vi "newTest_interface.vi"(0 "Daten":T1={"Report.lvclass"=refnum, "Norm"="", "last State"=enum."Initialize", "Norm ID"=0, "parameter"=[], "EMTestCWS500N.lvclass"=refnum, "CEG4500.lvclass"=refnum, "Tektronix RSA5106A.lvclass"=refnum, "erfolgreich"=FALSE, "log"="", "Kommentar"="", "Device Enum"=enum."emTestCWS500N", "Test Enum"=enum."HF-Felder", "debug"=FALSE, "tab"=enum."Hauptmenü", "ESD Pistol.lvclass"=refnum, "SubPnl Refnum"=refnum, "TabCtl Refnum"=refnum, "ButtonsEinblenden?"=FALSE}, 1 "Test in":refnum<class "Test.lvclass">, 3 "error in (no error)":errorcluster, 4 "VI Refnum":refnum<vi>) -> (7 "Test.lvclass":refnum<class "Test.lvclass">, 8 "abbrechen":bool, 10 "error out":errorcluster)   [LabVIEW 2013]
uses:
  Main/controls/Data.ctl
  classes/Datastructure/Report/Report.lvclass
  classes/Devices/emTestCWS500N/EMTestCWS500N.lvclass
  classes/Devices/CEG4500/CEG4500.lvclass
  classes/Devices/Tektronix RSA5106A/Tektronix RSA5106A.lvclass
  ESD Pistol.lvclass
  Main/controls/State.ctl
  classes/Devices/DeviceInterface/Devices.ctl
  classes/Tests/TestInterface/Tests.ctl
  Tabs.ctl
  classes/Datastructure/Test/Test.lvclass
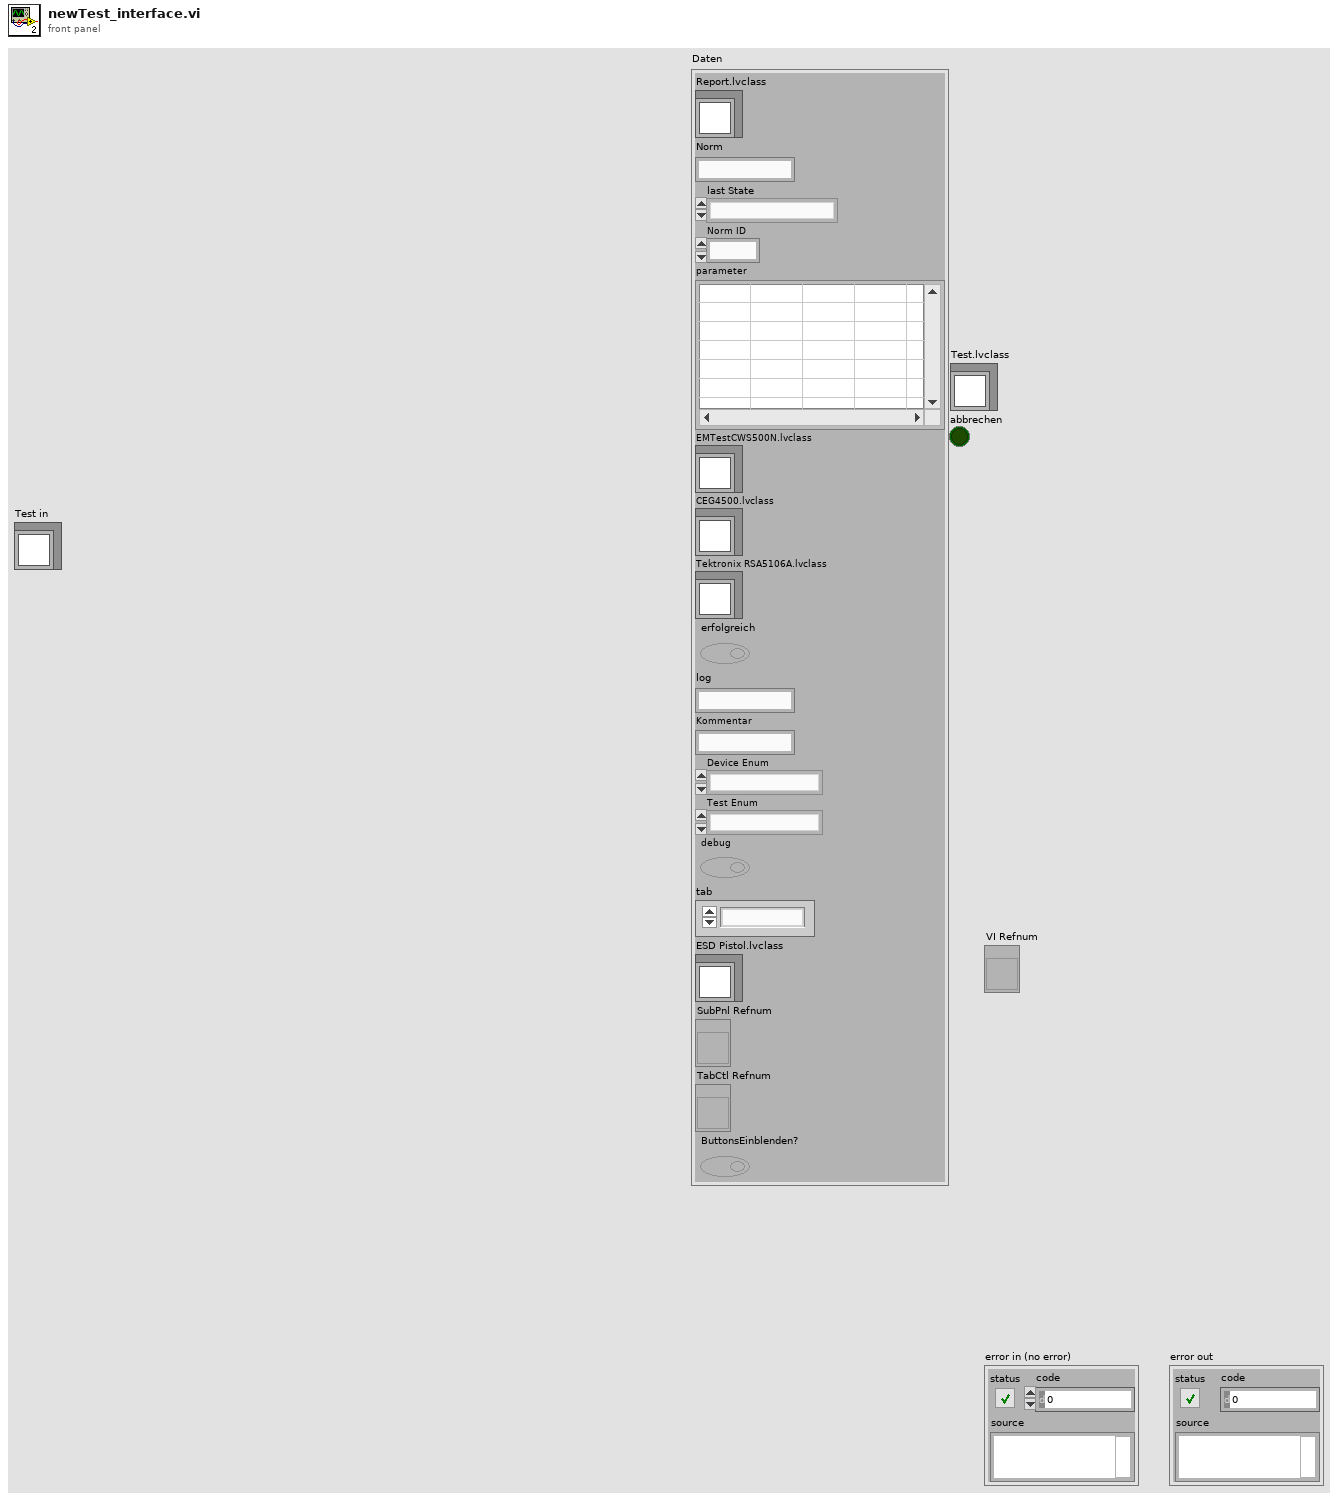
[diagram p1: front panel]
types:
  T1 = typedef "Data.ctl" = cluster{"Report.lvclass":refnum<class "Report.lvclass">, "Norm":string, "last State":T2, "Norm ID":i32, "parameter":string[][], "EMTestCWS500N.lvclass":refnum<class "EMTestCWS500N.lvclass">, "CEG4500.lvclass":refnum<class "CEG4500.lvclass">, "Tektronix RSA5106A.lvclass":refnum<class "Tektronix RSA5106A.lvclass">, "erfolgreich":bool, "log":string, "Kommentar":string, "Device Enum":T3, "Test Enum":T4, "debug":bool, "tab":T5, "ESD Pistol.lvclass":refnum<class "ESD Pistol.lvclass">, "SubPnl Refnum":refnum<vi>, "TabCtl Refnum":refnum<vi>, "ButtonsEinblenden?":bool}
  T2 = typedef "State.ctl" = enum16{"create Pdf", "load Report", "save Report", "do Test", "CDN Kalibrierung", "enter Report Parameters", "new Test", "Protokoll", "read Tree", "update Tree", "Fehler", "Initialize", "Wait for Event", "Exit"}
  T3 = typedef "Devices.ctl" = enum16{"unbekannt", "ESD Pistol", "Tektronix RSA5106A", "emTestCWS500N", "CEG-4500"}
  T4 = typedef "Tests.ctl" = enum16{"unbekannt", "Störaussendung", "Burst", "ESD", "Surge", "Spannungseinbruch", "HF-Felder"}
  T5 = typedef "Tabs.ctl" = enum32{"Hauptmenü", "Prüfbericht", "Einstellungen"}
  T6 = enum32{"Hauptmenü", "Prüfbericht", "Einstellungen"}
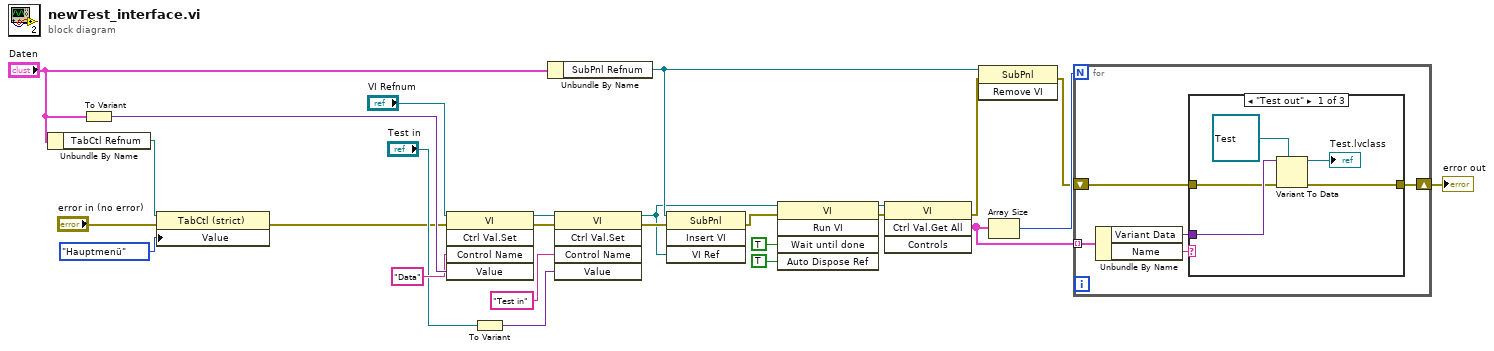
[diagram p0: block diagram]
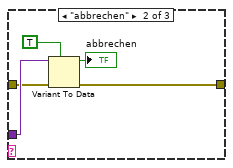
[diagram p2: hidden frame]
diagram:
  n1 = Unbundle By Name("Daten") -> ("TabCtl Refnum"=w12:refnum<vi>)
  n2 = To Variant(anything="Daten") -> (Variant=w16:variant)
  n3 = property class="TabCtl (strict)"(reference=w12, error in="error in (no error)", "Value"=T6."Hauptmenü") -> (error out=w1:errorcluster)  [unwired: 1 out]
  n4 = invoke class="VI" method="Ctrl Val.Set"(reference="VI Refnum", error in=w1, "Control Name"="Data", "Value"=w16) -> (reference out=w8:refnum<vi>, error out=w7:errorcluster)  [unwired: 1 in, 3 out]
  n5 = To Variant(anything="Test in") -> (Variant=w2:variant)
  n6 = Unbundle By Name("Daten") -> ("SubPnl Refnum"=w13:refnum<vi>)
  n7 = invoke class="VI" method="Ctrl Val.Set"(reference=w8, error in=w7, "Control Name"="Test in", "Value"=w2) -> (reference out=w5:refnum<vi>, error out=w6:errorcluster)  [unwired: 1 in, 3 out]
  n8 = invoke on="Invoke Node" class="SubPnl" method="Insert VI"(reference=w13, error in=w6, "VI Ref"=w5) -> (error out=w24:errorcluster)  [unwired: 1 in, 3 out]
  n9 = invoke on="Methodenknoten" class="VI" method="Run VI"(reference=w5, error in=w24, "Wait until done"=TRUE ("Warten bis beendet"), "Auto Dispose Ref"=TRUE ("Referenz automatisch schließen")) -> (reference out=w26:refnum<vi>, error out=w25:errorcluster)  [unwired: 1 in, 3 out]
  n10 = invoke class="VI" method="Ctrl Val.Get All"(reference=w26, error in=w25) -> (error out=w19:errorcluster, "Get All Control Values Variant"=w21:cluster{"Name":string, "Variant Data":variant}[])  [unwired: 2 in, 2 out]
  n11 = invoke on="Invoke Node" class="SubPnl" method="Remove VI"(reference=w13, error in=w19) -> (error out=w18:errorcluster)  [unwired: 1 in, 2 out]
  n12 = Array Size(array=w21) -> (size(s)=w20:i32)
  n13 = for {
    N: w20 -> [_]
    tunnel: w21 -> [w31] mode=indexing
    shift-right: [w27] -> w17
    shift-left: w18 -> [w28]
    n14 = Unbundle By Name(w31) -> ("Variant Data"=w29:variant, "Name"=w30:string)
    n15 = case shown="\"Test out\"" w30 {
      tunnel: w29 -> [w36 w41 _]
      tunnel: w28 -> [w35 w40 w42]
      tunnel: [w34 w39 w42] -> w27
      frame "Test out" {
        n16 = Variant To Data(error in=w35, type=refnum<class "Test.lvclass"> refnum ("Test.lvclass 2"), Variant=w36) -> (data=→"Test.lvclass":refnum<class "Test.lvclass">, error out=w34:errorcluster)
      }
      frame "abbrechen" {
        n17 = Variant To Data(error in=w40, type=TRUE ("Referenz automatisch schließen"), Variant=w41) -> (data=→"abbrechen":bool, error out=w39:errorcluster)
      }
      frame Default {
      }
    }
  }
  "error out" <- w17
